vi "交替背景色显示、缓冲添加项目.vi"() -> ()   [LabVIEW 2012, in "Listbox Tool.lvlib"]
uses:
  Listbox Tool.lvlib
  Method/Alternate BG Color.vi
  Method/Add Item Buffered.vi
panel:
  in  "停止按钮":bool
  in  "列表框":i32(listbox)=1
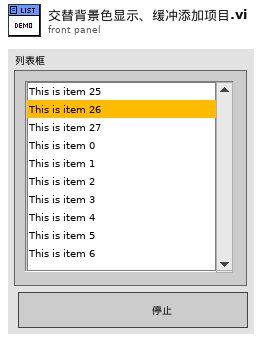
[diagram p1: front panel]
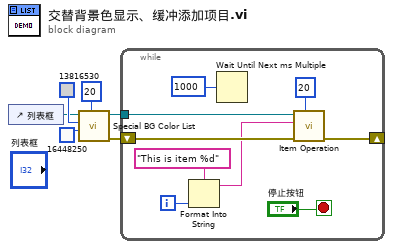
[diagram p0: block diagram]
diagram:
  n1 = control-ref of="列表框"() -> (w1:refnum<vi>)
  n2 = call-poly "Special BG Color List.vi"("Number of Rows"=20, "Second BG Color"=u32 16448250, "First BG Color"=u32 13816530, "Listbox Ref"=w1) -> ("错误输出"=w2:errorcluster, "Dup Listbox Ref"=w3:refnum<vi>)  [unwired: 6 in]
  n3 = while {
    tunnel: w3 -> [w15]
    shift-right: [w13] -> _
    shift-left: w2 -> [w14]
    i -> [w10]
    stop <- "停止按钮" stop-if-true
    n4 = Format Into String(format string="This is item %d" ("格式字符串"), w10) -> (resulting string=w8:string)  [unwired: 2 in, 1 out]
    n5 = Wait Until Next ms Multiple(millisecond multiple=u32 1000 ("毫秒倍数")) -> ()  [unwired: 1 out]
    n6 = call-poly "Item Operation.vi"("Items Array Length"=20, "错误输入"=w14, "Item"=w8, "Listbox Ref"=w15) -> ("错误输出"=w13:errorcluster)  [unwired: 6 in, 1 out]
  }
